vi "count.vi"(9 "nums":i32[](array[numeric]), 10 "cfg":string, 11 "cache":refnum<data-value>) -> (0 "count":u64)   [LabVIEW 2023, in "d12.lvlib"]
uses:
  d12.lvlib
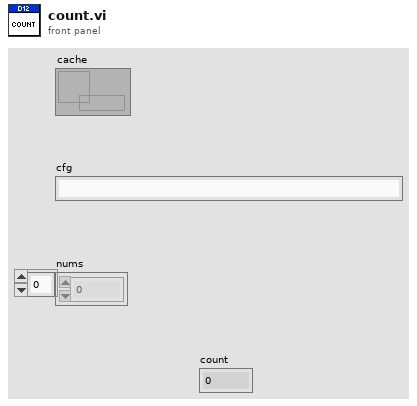
[diagram p1: front panel]
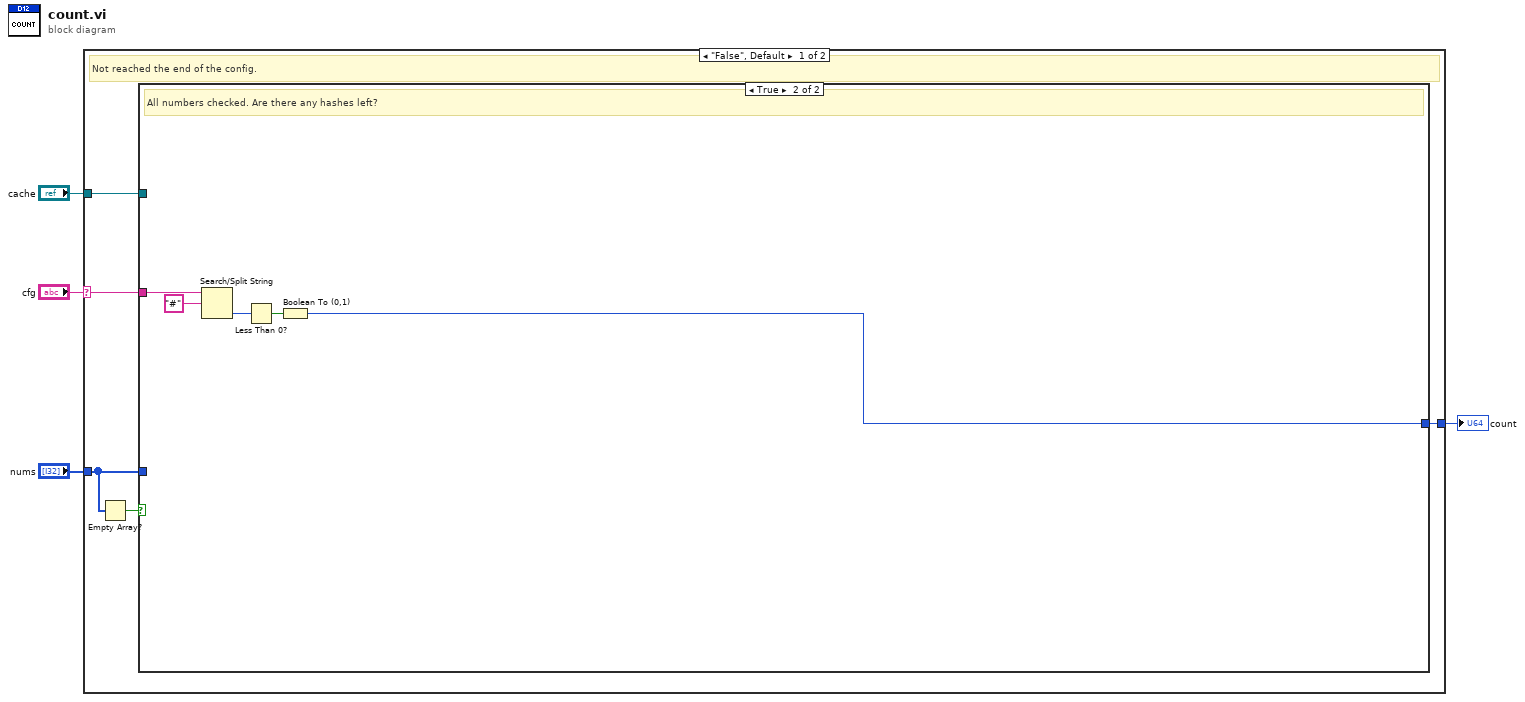
[diagram p0: block diagram]
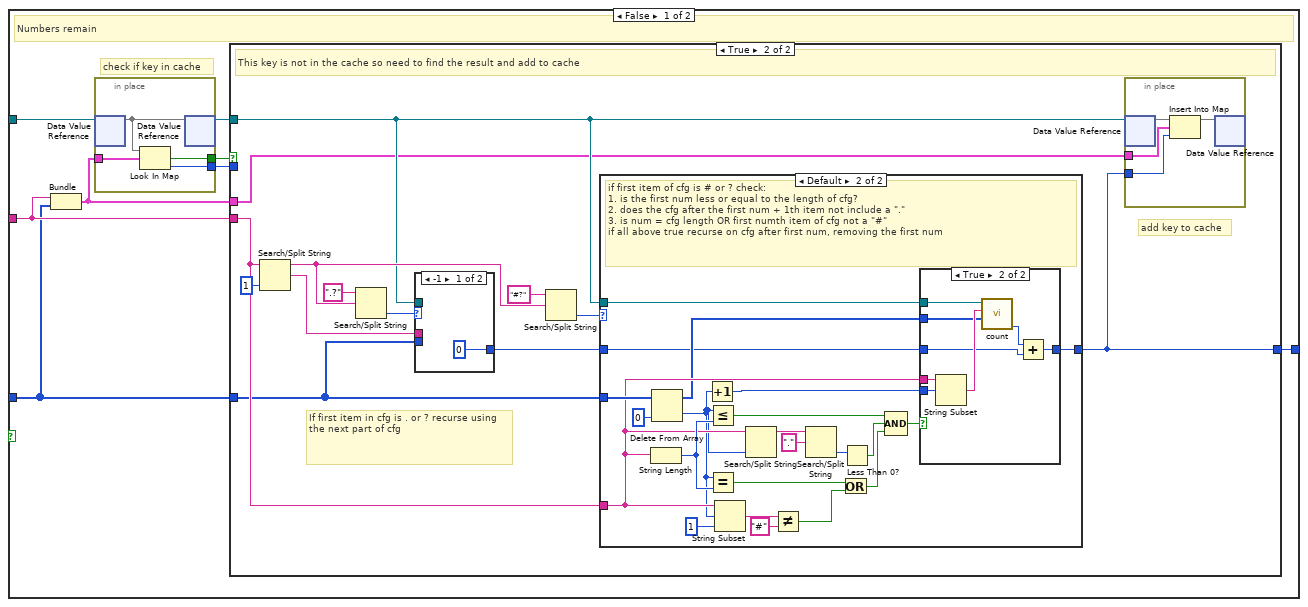
[diagram p2: hidden frame]
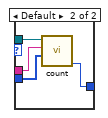
[diagram p6: hidden frame]
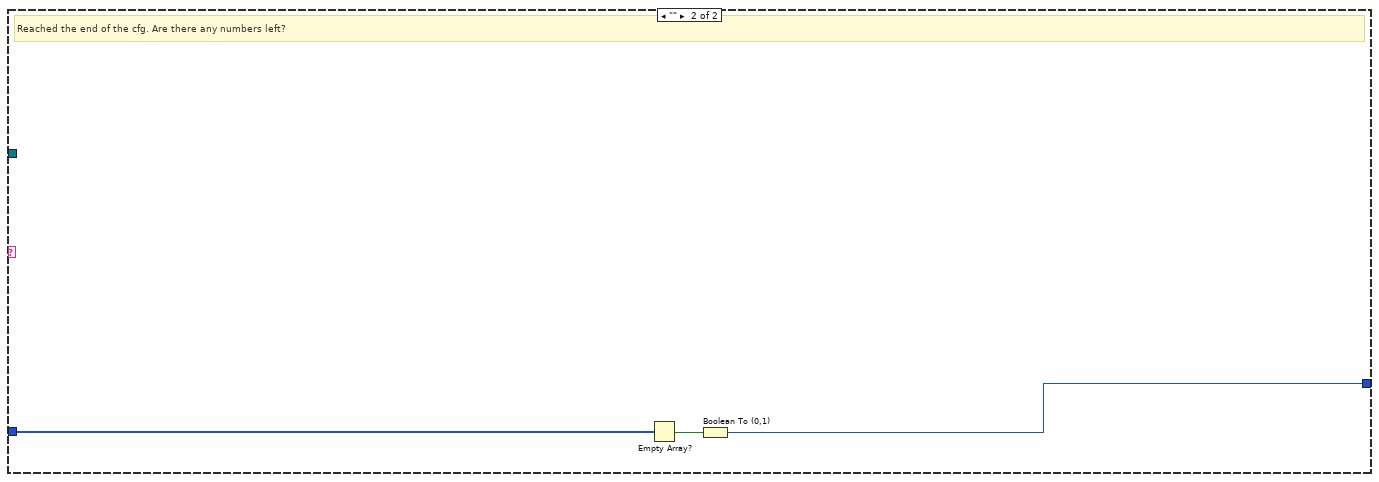
[diagram p7: hidden frame]
diagram:
  n1 = case shown="\"False\", Default" "cfg" {
    selector: "cfg" -> [w7 _]
    tunnel: "nums" -> [w6 w84]
    tunnel: [w8 w82] -> w1
    tunnel: "cache" -> [w5 _]
    frame "False", Default {
      # "Not reached the end of the config."
      n2 = Empty Array?(array=w6) -> (empty?=w9:bool)
      n3 = case shown="True" w9 {
        tunnel: w7 -> [w12 w81]
        tunnel: w6 -> [w11 _]
        tunnel: [w14 w77] -> w8
        tunnel: w5 -> [w17 _]
        frame False {
          # "check if key in cache"
          # "Numbers remain"
          n4 = Bundle(w12, "nums"=w11) -> (w10:cluster{string, "nums":i32[]})  [unwired: 1 in]
          n5 = in-place {
            in-place-border: w10 -> [w75]
            in-place-border: [w74] -> w15
            in-place-border: [w73] -> w16
            n6 = in-place-dvr #1(w17) -> (w76:map{cluster{string, "nums":i32[]}, u64})  [unwired: 1 out]
            n7 = Look In Map(map=w76, key=w75) -> (key not found?=w73:bool, value=w74:u64)  [unwired: 1 in]
            n8 = in-place-dvr #1(w76) -> (w13:refnum<data-value>)  [unwired: 1 out]
          }
          n9 = case shown="True" w16 {
            tunnel: w15 -> [w18 _]
            tunnel: [w18 w20] -> w14
            tunnel: w13 -> [_ w21]
            tunnel: w12 -> [_ w23]
            tunnel: w11 -> [_ w22]
            tunnel: w10 -> [_ w19]
            frame False {
              # "Key is in the cache, get the result."
            }
            frame True {
              # "add key to cache"
              # "If first item in cfg is . or ? recurse using the next part of cfg"
              # "This key is not in the cache so need to find the result and add to cache"
              n10 = Search/Split String(string=w23, offset (0)=1) -> (substring before match=w25:string, match + rest of string=w28:string)  [unwired: 1 in, 1 out]
              n11 = Search/Split String(string=".?", search string/char (-)=w25) -> (offset of match=w29:i32)  [unwired: 1 in, 2 out]
              n12 = case shown="-1" w29 {
                tunnel: w21 -> [_ w72]
                tunnel: w28 -> [_ w71]
                tunnel: w22 -> [_ w70]
                tunnel: [u64 0 ("count") w69] -> w27
                frame -1 {
                }
                frame Default {
                  n13 = call "count.vi"("nums"=w70, "cfg"=w71, "cache"=w72) -> ("count"=w69:u64)  [unwired: 8 in]
                }
              }
              n14 = Search/Split String(string="#?", search string/char (-)=w25) -> (offset of match=w24:i32)  [unwired: 1 in, 2 out]
              n15 = case shown="Default" w24 {
                tunnel: w21 -> [_ w58]
                tunnel: w27 -> [w36 w40]
                tunnel: [w36 w39] -> w20
                tunnel: w23 -> [_ w44]
                tunnel: w22 -> [_ w45]
                frame -1 {
                }
                frame Default {
                  # "if first item of cfg is # or ? check:\n1. is the first num less or equal to the length of cfg?\n2. does the cfg after the first num + 1th item not include a \".\"\n3. is num = cfg length OR first numth item of cfg not a \"#\"\nif all above true recurse on cfg after first num, removing the first num"
                  n16 = String Length(string=w44) -> (length=w50:i32)
                  n17 = Delete From Array(array=w45, index=0) -> (deleted portion=w38:i32, array with subset deleted=w42:i32[])  [unwired: 1 in]
                  n18 = Increment(x=w38) -> (x+1=w37:i32)
                  n19 = Less Or Equal?(x=w38, y=w50) -> (x <= y?=w55:bool)
                  n20 = Equal?(x=w38, y=w50) -> (x = y?=w51:bool)
                  n21 = String Subset(string=w44, offset (0)=w38, length (rest)=1 ("length (rest)")) -> (substring=w48:string)
                  n22 = Search/Split String(string=w44, offset (0)=w38) -> (substring before match=w57:string)  [unwired: 1 in, 2 out]
                  n23 = Not Equal?(x=w48, y="#") -> (x != y?=w46:bool)
                  n24 = Search/Split String(string=w57, search string/char (-)=".") -> (offset of match=w54:i32)  [unwired: 1 in, 2 out]
                  n25 = Or(x=w51, y=w46) -> (x .or. y?=w52:bool)
                  n26 = Less Than 0?(x=w54) -> (x < 0?=w53:bool)
                  n27 = Compound Arithmetic op=AND(w55, w53, w52) -> (w41:bool)
                  n28 = case shown="True" w41 {
                    tunnel: w58 -> [_ w67]
                    tunnel: w44 -> [_ w66]
                    tunnel: w37 -> [_ w65]
                    tunnel: w42 -> [_ w63]
                    tunnel: w40 -> [w59 w60]
                    tunnel: [w59 w62] -> w39
                    frame False {
                    }
                    frame True {
                      n29 = String Subset(string=w66, offset (0)=w65) -> (substring=w64:string)  [unwired: 1 in]
                      n30 = call "count.vi"("nums"=w63, "cfg"=w64, "cache"=w67) -> ("count"=w61:u64)  [unwired: 8 in]
                      n31 = Add(x=w61, y=w60) -> (x+y=w62:u64)
                    }
                  }
                }
              }
              n32 = in-place {
                in-place-border: w19 -> [w33]
                in-place-border: w20 -> [w32]
                n33 = in-place-dvr #2(w21) -> (w35:map{cluster{string, "nums":i32[]}, u64})  [unwired: 1 out]
                n34 = Insert Into Map(map in=w35, key=w33, value=w32) -> (map out=w34:map{cluster{string, "nums":i32[]}, u64})  [unwired: 2 out]
                n35 = in-place-dvr #2(w34) -> ()  [unwired: 2 out]
              }
            }
          }
        }
        frame True {
          # "All numbers checked. Are there any hashes left?"
          n36 = Search/Split String(string=w81, search string/char (-)="#") -> (offset of match=w79:i32)  [unwired: 1 in, 2 out]
          n37 = Less Than 0?(x=w79) -> (x < 0?=w78:bool)
          n38 = Boolean To (0,1)(Boolean=w78) -> (0, 1=w77:i16)
        }
      }
    }
    frame "" {
      # "Reached the end of the cfg. Are there any numbers left?"
      n39 = Empty Array?(array=w84) -> (empty?=w83:bool)
      n40 = Boolean To (0,1)(Boolean=w83) -> (0, 1=w82:i16)
    }
  }
  "count" <- w1
